vi "Tree Data Types and XML Example.vi"(11 "Tree":string(tree)) -> (10 "XML String":string="<Parent MetaData=\"You can add descriptions to your trees.\">\n\n<Child>\n<Attr Name=\"MyInteger\" Type=\"Int\">\n12\n</Attr>\r\n<Attr Name=\"My1DInteger\" Type=\"1D Int\">\n23, 34\n</Attr>\r\n<Attr Name=\"My2DInteger\" Type=\"2D Int\">\n23, 34;\r\n45, 56\n</Attr>\r\n<Attr Name=\"MyPath\" Type=\"Path\">\n\"test.llb\"\n</Attr>\r\n<Attr Name=\"My1DPath\" Type=\"1D Path\">\n\"test.llb\", \"\\\\netpath\\\"\n</Attr>\r\n<Attr Name=\"My2DPath\" Type=\"2D Path\">\n\"test.llb\", \"\\\\netpath\\\";\r\n\"a\", \"b\"\n</Attr>\r\n<Attr Name=\"MyBool\" Type=\"Bool\">\nTRUE\n</Attr>\r\n<Attr Name=\"My1DBool\" Type=\"1D Bool\">\nTRUE, FALSE\n</Attr>\r\n<Attr Name=\"My2DBoolArray\" Type=\"2D Bool\">\nFALSE, TRUE;\r\nFALSE, TRUE\n</Attr>\r\n<Attr Name=\"MyFloat\" Type=\"Flt\">\n3.14\n</Attr>\r\n<Attr Name=\"My1DFloat\" Type=\"1D Flt\">\n9.8596, 97.211712\n</Attr>\r\n<Attr Name=\"My2DFloat\" Type=\"2D Flt\">\n9.8596, 97.211712;\r\n97.211712, 9450.116981\n</Attr>\r\n<Attr Name=\"MyString\" Type=\"String\" MetaData=\"Any Tree Data class can use this field.\">\n\"Foo\"\n</Attr>\r\n<Attr Name=\"My1DString\" Type=\"1D String\">\n\"Foo\", \"Bar\"\n</Attr>\r\n<Attr Name=\"My2DString\" Type=\"2D String\">\n\"Foo\", \"Bar\";\r\n\"Bar\", \"&lt;&gt;&apos;&quot;&amp;&semi;\"\n</Attr>\n\n</Child>\n</Parent>")   [LabVIEW 2020, in "NI_VIAnCFGDataStructure.lvlib" / "Tree.lvclass"]
uses:
  <vilib>/addons/analyzer/VIAnCFGDataStructure/Tree Manager/Tree.lvclass
  <vilib>/addons/analyzer/VIAnCFGDataStructure/Tree Manager/API/Set Meta Data.vi
  <vilib>/addons/analyzer/VIAnCFGDataStructure/Tree Manager/API/Set Attributes Tree Data.vi
  <vilib>/addons/analyzer/VIAnCFGDataStructure/Tree Manager/API/List Roots.vi
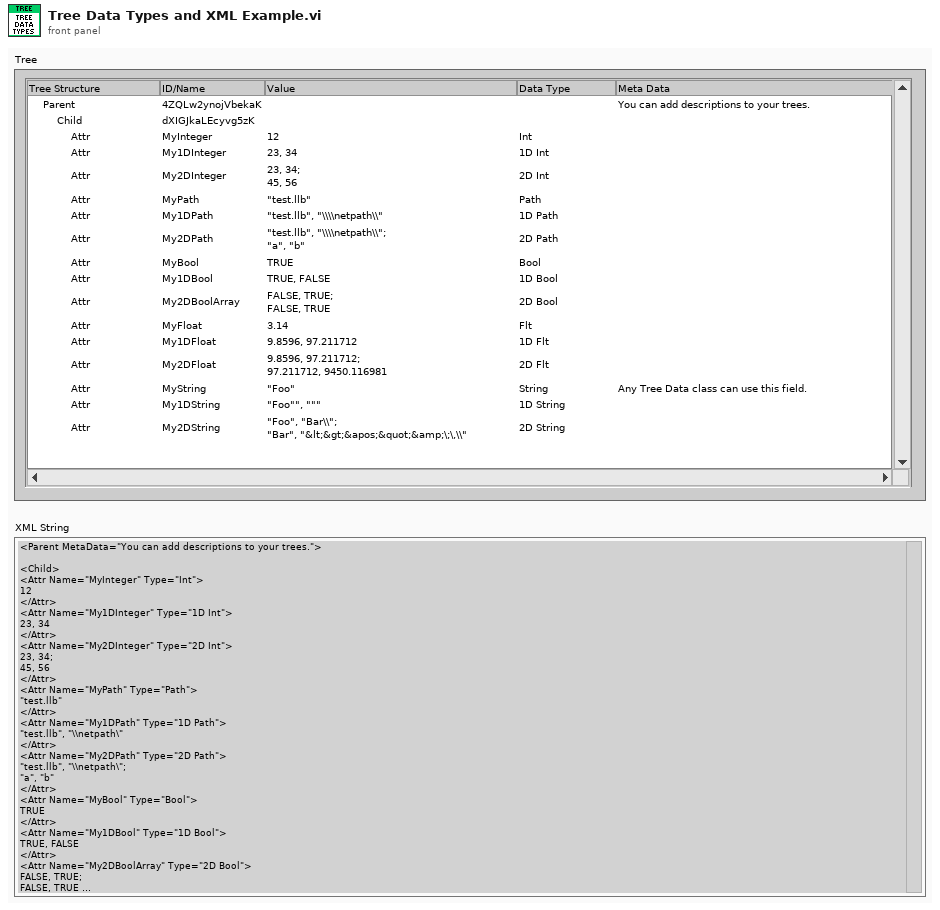
[diagram p1: front panel]
types:
  T1 = typedef "NI_VIAnCFGDataStructure.lvlib/Tree.lvclass/Session Handle.ctl" = refnum<data-value>
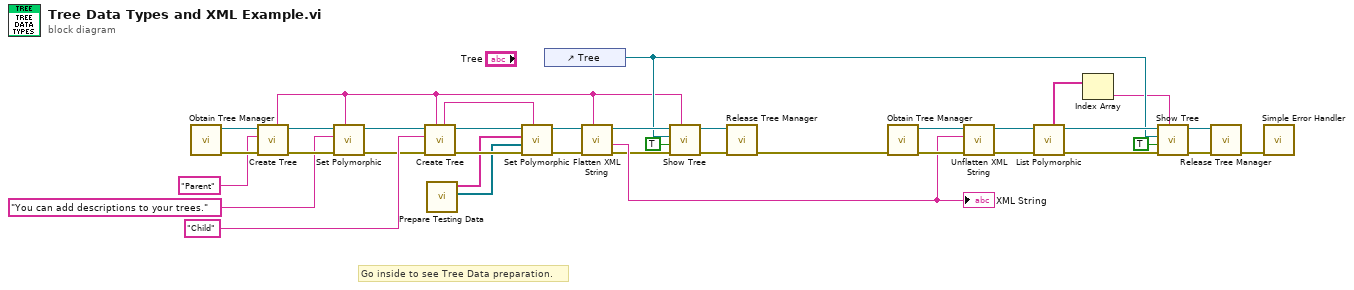
[diagram p0: block diagram]
diagram:
  # "Go inside to see Tree Data preparation."
  n1 = call <vilib>:"Obtain Tree Manager.vi"() -> ("Error Out"=w36:errorcluster, "Tree"=w37:T1)  [unwired: 10 in]
  n2 = call <vilib>:"Create Tree.vi"("Error In"=w36, "Name"="Parent", "Tree Manager"=w37) -> ("Error Out"=w11:errorcluster, "Tree Manager"=w15:T1, "Unique ID"=w14:string)  [unwired: 6 in]
  n3 = call-poly <vilib>:"Set Polymorphic.vi"("Tree ID"=w14, "Error In"=w11, "Meta Data"="You can add descriptions to your trees.", "Tree Manager"=w15) -> ("Error Out"=w12:errorcluster, "Tree Manager"=w13:T1)  [unwired: 6 in]
  n4 = call <vilib>:"Create Tree.vi"("Parent ID (empty)"=w14, "Error In"=w12, "Name"="Child", "Tree Manager"=w13) -> ("Error Out"=w32:errorcluster, "Tree Manager"=w33:T1, "Unique ID"=w8:string)  [unwired: 5 in]
  n5 = call <vilib>:"Prepare Testing Data.vi"() -> ("Attr Data"=w17:refnum<class "Tree Data.lvclass">[], "Attr Names"=w16:string[])  [unwired: 10 in]
  n6 = call-poly <vilib>:"Set Polymorphic.vi"("Tree ID"=w8, "Error In"=w32, "Attributes Values"=w17, "Attributes Names"=w16, "Tree Manager"=w33) -> ("Error Out"=w7:errorcluster, "Tree Manager"=w9:T1)  [unwired: 4 in, 1 out]
  n7 = control-ref of="Tree"() -> (w19:refnum<vi>)
  n8 = call <vilib>:"Flatten XML String.vi"("Root ID"=w14, "Error In"=w7, "Tree"=w9) -> ("Error Out"=w22:errorcluster, "XML String"=w24:string, "Tree"=w23:T1)  [unwired: 6 in]
  "XML String" <- w24
  n9 = call <vilib>:"Show Tree.vi"("Root ID"=w14, "Error In"=w22, "Show IDs (False)"=TRUE, "Tree Ref"=w19, "Tree"=w23) -> ("Error Out"=w21:errorcluster, "Tree"=w20:T1)  [unwired: 5 in]
  n10 = call <vilib>:"Release Tree Manager.vi"("Error In"=w21, "Tree"=w20) -> ("Error Out"=w6:errorcluster)  [unwired: 9 in]
  n11 = call <vilib>:"Obtain Tree Manager.vi"("Error In"=w6) -> ("Error Out"=w29:errorcluster, "Tree"=w30:T1)  [unwired: 9 in]
  n12 = call <vilib>:"Unflatten XML String.vi"("Error In"=w29, "XML String"=w24, "Tree"=w30) -> ("Error Out"=w27:errorcluster, "Tree"=w28:T1)  [unwired: 7 in]
  n13 = call-poly <vilib>:"List Polymorphic.vi"("Error In"=w27, "Tree"=w28) -> ("Error Out"=w25:errorcluster, "Tree"=w26:T1, "Roots IDs"=w18:string[])  [unwired: 6 in, 1 out]
  n14 = Index Array(array=w18) -> (element=w3:string)  [unwired: 1 in]
  n15 = call <vilib>:"Show Tree.vi"("Root ID"=w3, "Error In"=w25, "Show IDs (False)"=TRUE, "Tree Ref"=w19, "Tree"=w26) -> ("Error Out"=w4:errorcluster, "Tree"=w5:T1)  [unwired: 5 in]
  n16 = call <vilib>:"Release Tree Manager.vi"("Error In"=w4, "Tree"=w5) -> ("Error Out"=w31:errorcluster)  [unwired: 9 in]
  n17 = call <vilib>:"Simple Error Handler.vi"("error in (no error)"=w31) -> ()  [unwired: 4 in, 5 out]
